vi "get UI reference.vi"(8 "error in":errorcluster, 11 "set source separate in":refnum<class "set source separate.lvclass">) -> (0 "error out":errorcluster, 2 "VI Refnum":refnum<vi>, 3 "set source separate out":refnum<class "set source separate.lvclass">)   [LabVIEW 2013, in "set source separate.lvclass"]
uses:
  set source separate.lvclass
  source sep ui.vi
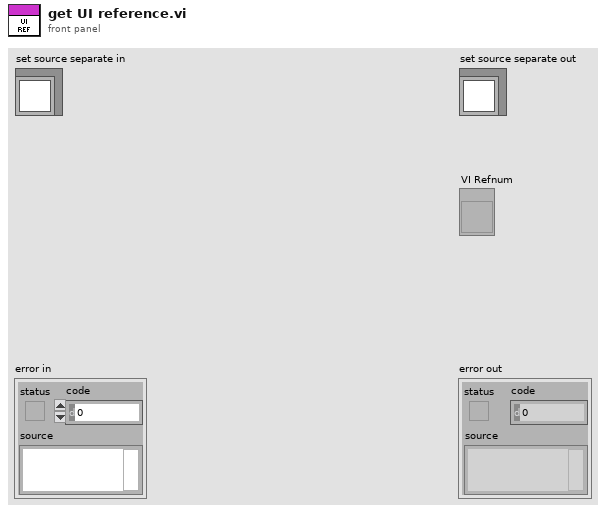
[diagram p1: front panel]
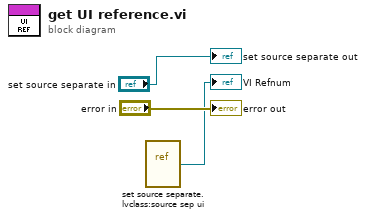
[diagram p0: block diagram]
diagram:
  n1 = vi-ref "set source separate.lvclass:source sep ui.vi"() -> (→"VI Refnum":refnum<vi>)
  "error out" <- "error in"
  "set source separate out" <- "set source separate in"
